vi "sha256.vi"(8 "error in (no error)":errorcluster, 11 "data_decoded":string) -> (0 "error out":errorcluster, 3 "data_encoded":string)   [LabVIEW 2015, in "lv-dropbox.lvlib" / "cryptography.lvlib"]
uses:
  cryptography.lvlib
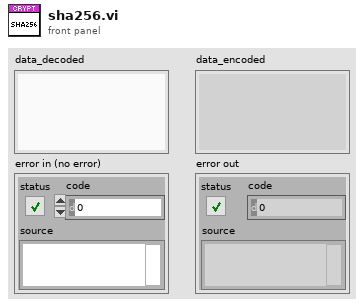
[diagram p1: front panel]
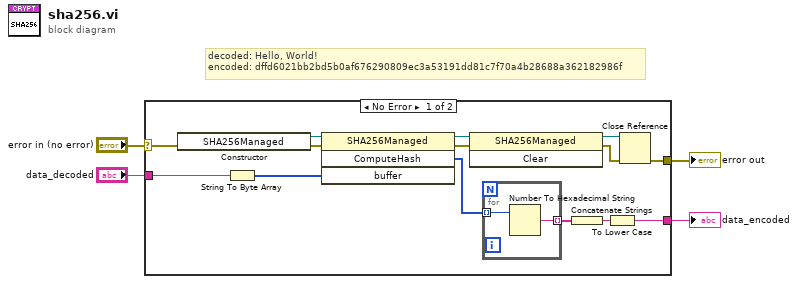
[diagram p0: block diagram]
diagram:
  # "decoded: Hello, World!\nencoded: dffd6021bb2bd5b0af676290809ec3a53191dd81c7f70a4b28688a362182986f"
  n1 = case shown="No Error" "error in (no error)" {
    selector: "error in (no error)" -> [w16 w21]
    tunnel: "data_decoded" -> [w18 _]
    tunnel: [w5 _] -> w2
    tunnel: [w13 w21] -> w1
    frame No Error {
      n2 = constructor class="SHA256Managed"(error in=w16) -> (reference out=w12:refnum<k24>, error out=w11:errorcluster)  [unwired: 2 in, 1 out]
      n3 = String To Byte Array(string=w18) -> (unsigned byte array=w17:u8[])
      n4 = invoke class="SHA256Managed" method="ComputeHash"(reference=w12, error in=w11, "buffer"=w17) -> (reference out=w10:refnum<k24>, error out=w9:errorcluster, "ComputeHash"=w8:u8[])  [unwired: 1 in, 1 out]
      n5 = invoke class="SHA256Managed" method="Clear"(reference=w10, error in=w9) -> (reference out=w15:refnum<k24>, error out=w14:errorcluster)  [unwired: 1 in, 1 out]
      n6 = for {
        tunnel: w8 -> [w20] mode=indexing
        tunnel: [w19] -> w7 mode=indexing
        n7 = Number To Hexadecimal String(2:w20) -> (0:w19:string)  [unwired: 1 in]
      }
      n8 = Concatenate Strings(w7) -> (w6:string)
      n9 = To Lower Case(string=w6) -> (all lower case string=w5:string)
      n10 = Close Reference(reference=w15, error in (no error)=w14) -> (error out=w13:errorcluster)
    }
    frame Error {
    }
  }
  "error out" <- w1
  "data_encoded" <- w2
